vi "FTW-Test-TagActor.vi"() -> ()   [LabVIEW 2015]
uses:
  source/actor/Connector/FTW-ActorConnector.lvclass
panel:
  out "String 2":string
  out "String":string
  out "error out":errorcluster
  out "Response":string
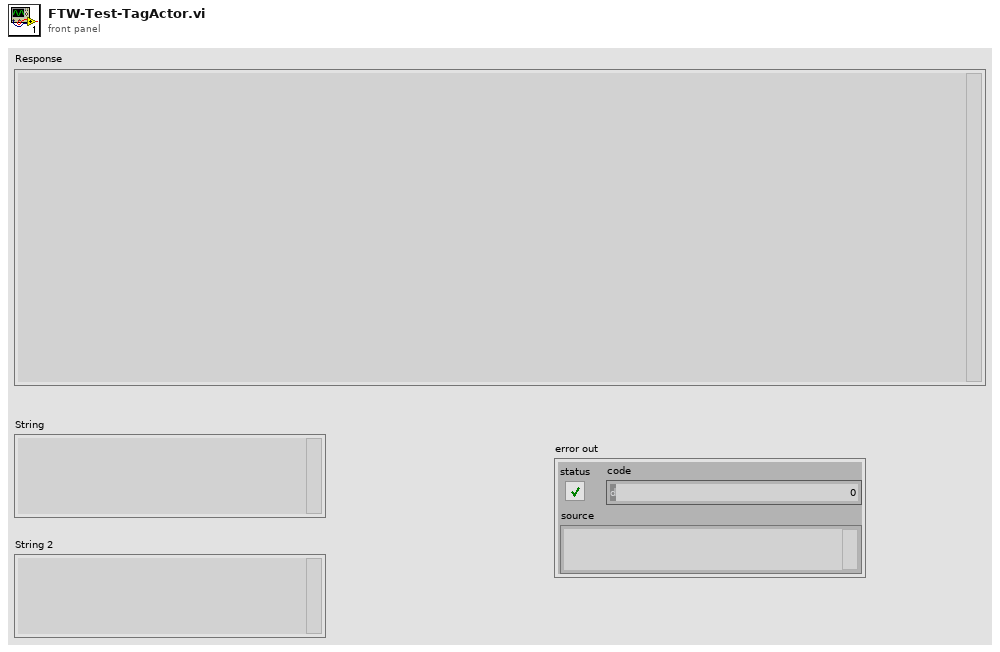
[diagram p1: front panel]
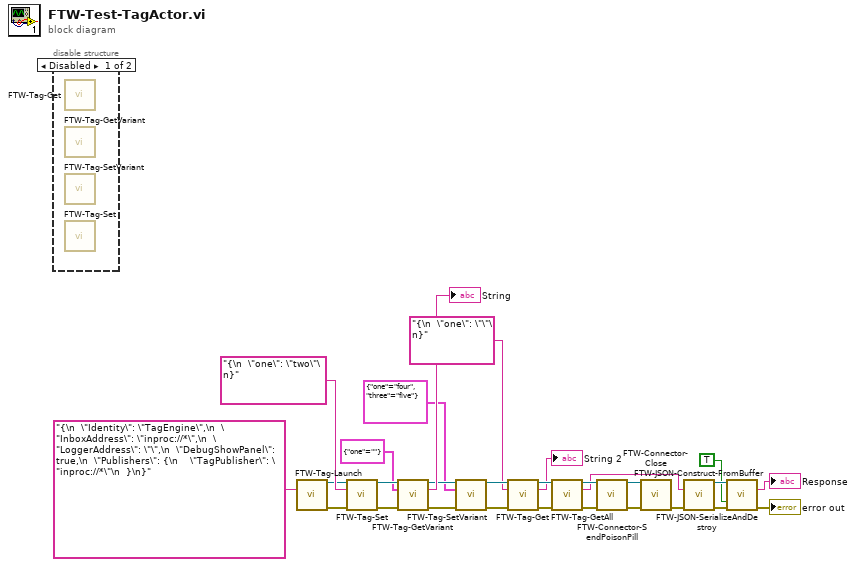
[diagram p0: block diagram]
diagram:
  n1 = disable-structure shown="Disabled" {
    frame Disabled {
      n2 = call "FTW-Tag-Get.vi"() -> ()  [unwired: 12 in, 4 out]
      n3 = call "FTW-Tag-GetVariant.vi"() -> ()  [unwired: 12 in, 4 out]
      n4 = call "FTW-Tag-SetVariant.vi"() -> ()  [unwired: 13 in, 3 out]
      n5 = call "FTW-Tag-Set.vi"() -> ()  [unwired: 13 in, 3 out]
    }
    frame Enabled {
    }
  }
  n6 = call "FTW-Tag-Launch.vi"("FTW Tag Configuration"="{\n  \"Identity\": \"TagEngine\",\n  \"InboxAddress\": \"inproc://*\",\n  \"LoggerAddress\": \"\",\n  \"DebugShowPanel\": true,\n  \"Publishers\": {\n    \"TagPublisher\": \"inproc://*\"\n  }\n}") -> ("FTW Tag Connector"=w15:refnum<class "FTW-ActorConnector.lvclass">, "error out"=w14:errorcluster)  [unwired: 11 in, 2 out]
  n7 = call "FTW-Tag-Set.vi"("FTW Actor Connector In"=w15, "Tag Object"="{\n  \"one\": \"two\"\n}" ("FTW Tag Configuration"), "error in (no error)"=w14) -> ("FTW Actor Connector"=w11:refnum<class "FTW-ActorConnector.lvclass">, "error out"=w19:errorcluster)  [unwired: 10 in, 1 out]
  n8 = call "FTW-Tag-GetVariant.vi"("FTW Actor Connector In"=w11, "Tag Object"=cluster{"one":string} {"one"=""}, "error in (no error)"=w19) -> ("FTW Actor Connector"=w7:refnum<class "FTW-ActorConnector.lvclass">, "Response"=→"String":string, "error out"=w12:errorcluster)  [unwired: 9 in, 1 out]
  n9 = call "FTW-Tag-SetVariant.vi"("FTW Actor Connector In"=w7, "Tag Object"=cluster{"one":string, "three":string} {"one"="four", "three"="five"}, "error in (no error)"=w12) -> ("FTW Actor Connector"=w4:refnum<class "FTW-ActorConnector.lvclass">, "error out"=w8:errorcluster)  [unwired: 10 in, 1 out]
  n10 = call "FTW-Tag-Get.vi"("FTW Actor Connector In"=w4, "Tag Object"="{\n  \"one\": \"\"\n}" ("FTW Tag Configuration"), "error in (no error)"=w8) -> ("FTW Actor Connector"=w3:refnum<class "FTW-ActorConnector.lvclass">, "Response"=→"String 2":string, "error out"=w5:errorcluster)  [unwired: 9 in, 1 out]
  n11 = call "FTW-Tag-GetAll.vi"("FTW Actor Connector In"=w3, "error in (no error)"=w5) -> ("FTW Actor Connector"=w16:refnum<class "FTW-ActorConnector.lvclass">, "Response"=w13:string, "error out"=w17:errorcluster)  [unwired: 10 in, 1 out]
  n12 = call-dynamic "FTW-Connector-SendPoisonPill.vi"("FTW Actor Connector"=w16, "error in"=w17) -> ("FTW Actor Connector out"=w27:refnum<class "FTW-ActorConnector.lvclass">, "error out"=w26:errorcluster)  [unwired: 8 in, 4 out]
  n13 = call-dynamic "FTW-Connector-Close.vi"("FTW Actor Connector"=w27, "error in"=w26) -> ("error out"=w25:errorcluster)  [unwired: 13 in]
  n14 = call "FTW-JSON-Construct-FromBuffer.vi"("JSON String (UTF-8)"=w13, "error in"=w25) -> ("JSON"=w22:refnum<class "FTW-Container.lvclass">, "error out"=w24:errorcluster)  [unwired: 12 in]
  n15 = call "FTW-JSON-SerializeAndDestroy.vi"("JSON"=w22, "Pretty Print"=TRUE, "error in"=w24) -> ("JSON String (UTF-8)"=→"Response":string, "error out"=→"error out":errorcluster)  [unwired: 11 in]
